vi "sv_Shift and Low Pass Filter (N Ch WDT) with IC.vi"(0 "input signals":waveform(dbl)[](array[waveform]), 1 "reset? (F)":bool, 7 "center":dbl, 9 "decimation factor":i32, 12 "initial conditions":T2 {"filter settings"."filters"."coefficients" format="%.2f"}, 13 "new dt":dbl) -> (4 "enveloped signals":waveform(dbl)[](array[waveform]), 14 "final conditions":T2 {"filter settings"."filters"."coefficients" format="%.2f"})   [LabVIEW 2017, in "SoundVib_FaultAnalysis.lvlib"]
uses:
  <vilib>/addons/Sound and Vibration/Order Analysis/Fault Analysis/SoundVib_FaultAnalysis.lvlib
  <vilib>/addons/_NISVFA/_Shared subVIs/Controls/OAT Decimation Filter.ctl
  <vilib>/addons/Sound and Vibration/Order Analysis/Resample Order Tracking/SubVIs/OAT Frequency Shift (Mixer).vi
  <vilib>/addons/Sound and Vibration/Order Analysis/Resample Order Tracking/SubVIs/oa_Decimation with CIC and Compensation Filter.vi
  <vilib>/addons/Sound and Vibration/Order Analysis/Fault Analysis/SubVIs/oa_Demodulation Initial States (1 Channel).vi
  <vilib>/addons/Sound and Vibration/Order Analysis/Adv Resampling/OAT Single Stage Decimation with IC.vi
  <vilib>/addons/Sound and Vibration/Order Analysis/Resample Order Tracking/SubVIs/OAT CIC Decimation.vi
  <vilib>/addons/Sound and Vibration/Order Analysis/Resample Order Tracking/SubVIs/oa_Interpolate Zeros Between Samples.vi
  <vilib>/addons/Sound and Vibration/Order Analysis/Resample Order Tracking/SubVIs/oa_Calculate Delay of CIC Decimation Interpolation Filter.vi
  <vilib>/addons/Sound and Vibration/Order Analysis/Resample Order Tracking/SubVIs/oa_Create CIC Compensation Filter.vi
  <vilib>/addons/Sound and Vibration/Order Analysis/Resample Order Tracking/SubVIs/oa_Create CIC LP Truncation Filter.vi
  <vilib>/addons/Sound and Vibration/Order Analysis/Resample Order Tracking/SoundVib_Resampling.lvlib
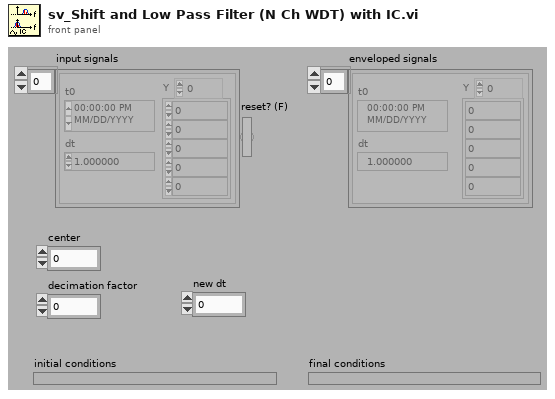
[diagram p1: front panel]
types:
  T1 = typedef "OAT Decimation Filter.ctl" = cluster{"coefficients":dbl[], "factor":i32}
  T2 = cluster{"filter settings":cluster{"CIC Settings":cluster{"Numeric":i32, i32, i32}, "filters":T1[], "delay":i32, "interpolation factor":i32}, "filter states":cluster{"t0":dbl, "phase":dbl, "real filter state":cluster{cluster{dbl[]}, cluster{dbl[]}[]}, "imaginary filter state":cluster{cluster{dbl[]}, cluster{dbl[]}[]}, "delay":i32}[], "reset pending":bool}
  T3 = cluster{"t0":dbl, "phase":dbl, "real filter state":cluster{cluster{dbl[]}, cluster{dbl[]}[]}, "imaginary filter state":cluster{cluster{dbl[]}, cluster{dbl[]}[]}, "delay":i32}[]
  T4 = cluster{"t0":dbl, "phase":dbl, "real filter state":cluster{cluster{dbl[]}, cluster{dbl[]}[]}, "imaginary filter state":cluster{cluster{dbl[]}, cluster{dbl[]}[]}, "delay":i32}
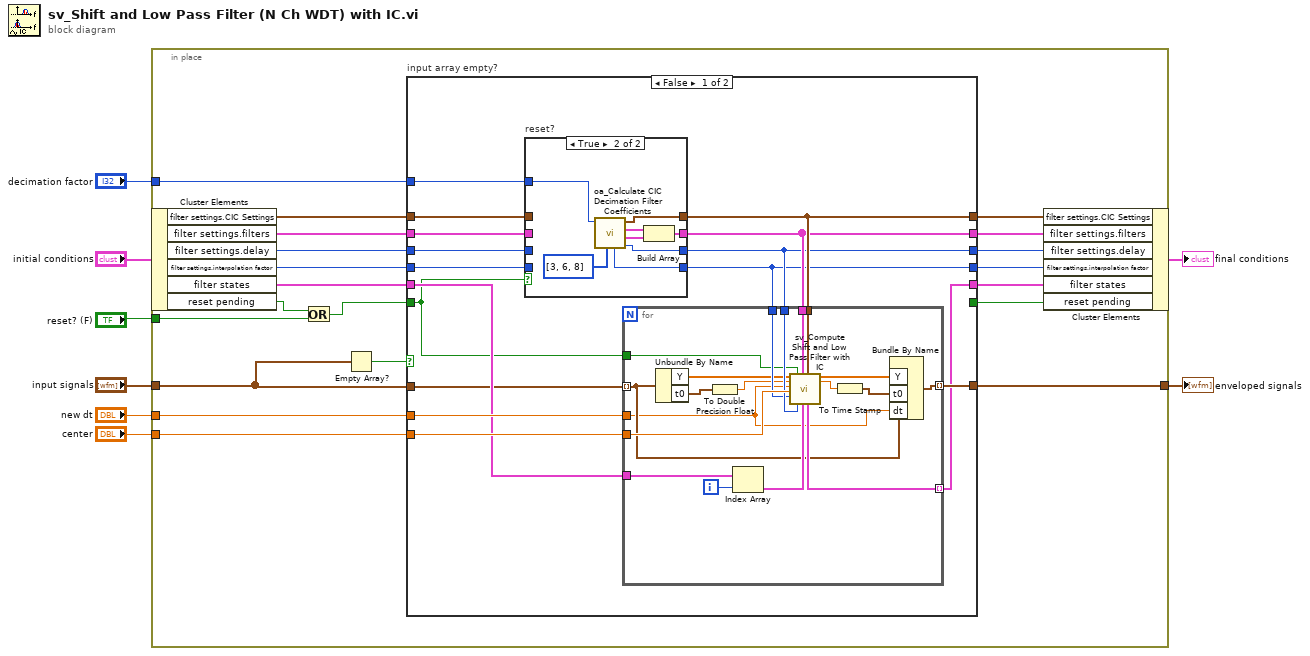
[diagram p0: block diagram]
diagram:
  n1 = in-place {
    in-place-border: "input signals" -> [w9]
    in-place-border: "decimation factor" -> [w28]
    in-place-border: "center" -> [w27]
    in-place-border: "new dt" -> [w26]
    in-place-border: "reset? (F)" -> [w13]
    in-place-border: [w25] -> w1
    n2 = in-place-cluster #1("initial conditions") -> ("filter settings.CIC Settings"=w22:cluster{"Numeric":i32, i32, i32}, "filter settings.filters"=w21:T1[], "filter settings.delay"=w20:i32, "filter settings.interpolation factor"=w19:i32, "filter states"=w24:T3, "reset pending"=w14:bool)
    n3 = Or(x=w14, y=w13) -> (x .or. y?=w12:bool)
    n4 = Empty Array?(array=w9) -> (empty?=w11:bool)
    n5 = case "input array empty?" shown="False" w11 {
      tunnel: w28 -> [w44 _]
      tunnel: w27 -> [w43 _]
      tunnel: w26 -> [w42 _]
      tunnel: [w41 w76] -> w25
      tunnel: w24 -> [w40 w77]
      tunnel: [w39 w77] -> w23
      tunnel: w22 -> [w38 w81]
      tunnel: w21 -> [w37 w80]
      tunnel: w20 -> [w36 w79]
      tunnel: w19 -> [w35 w78]
      tunnel: [w34 w81] -> w18
      tunnel: [w33 w80] -> w17
      tunnel: [w32 w79] -> w16
      tunnel: [w31 w78] -> w15
      tunnel: w12 -> [w30 w82]
      tunnel: [_ w82] -> w10
      tunnel: w9 -> [w29 w76]
      frame False {
        n6 = case "reset?" shown="True" w30 {
          tunnel: [w67 w75] -> w34
          tunnel: [w66 w72] -> w33
          tunnel: [w64 w71] -> w31
          tunnel: [w65 w70] -> w32
          tunnel: w44 -> [_ w69]
          tunnel: w38 -> [w67 _]
          tunnel: w37 -> [w66 _]
          tunnel: w36 -> [w65 _]
          tunnel: w35 -> [w64 _]
          frame False {
          }
          frame True {
            n7 = call <vilib>:"oa_Calculate CIC Decimation Filter Coefficients.vi"("CIC stages"=i32[] [3, 6, 8], "decimation/interpolation factor"=w69) -> ("delay"=w70:i32, "lp filter settings"=w73:T1, "compensation filter settings"=w74:T1, "CIC Settings"=w75:cluster{"Numeric":i32, i32, i32}, "interpolation factor"=w71:i32)  [unwired: 5 in]
            n8 = Build Array(w74, w73) -> (w72:T1[])
          }
        }
        n9 = for {
          tunnel: w43 -> [w63]
          tunnel: w42 -> [w50]
          tunnel: [w47] -> w41 mode=indexing
          tunnel: w40 -> [w58]
          tunnel: [w62] -> w39 mode=indexing
          tunnel: w34 -> [w45]
          tunnel: w33 -> [w46]
          tunnel: w32 -> [w61]
          tunnel: w31 -> [w60]
          tunnel: w30 -> [w59]
          tunnel: w29 -> [w54] mode=indexing
          i -> [w57]
          n10 = Unbundle By Name(w54) -> ("Y"=w55:dbl[], "t0"=w52:timestamp)
          n11 = To Double Precision Float(number=w52) -> (double precision float=w51:dbl)
          n12 = Index Array(array=w58, index=w57) -> (element=w56:T4)
          n13 = call <vilib>:"sv_Compute Shift and Low Pass Filter with IC.vi"("input signal"=w55, "t0"=w51, "new dt"=w50, "center"=w63, "interpolation factor"=w60, "reset? (F)"=w59, "delay"=w61, "filters"=w46, "initial conditions"=w56, "CIC settings"=w45) -> ("final conditions"=w62:T4, "enveloped signal"=w53:dbl[], "t0 out"=w49:dbl)  [unwired: 6 in, 1 out]
          n14 = To Time Stamp(1:w49) -> (0:w48:timestamp)
          n15 = Bundle By Name(cluster=w54, "Y"=w53, "t0"=w48, "dt"=w50) -> (w47:waveform(dbl))
        }
      }
      frame True {
      }
    }
    n16 = in-place-cluster #1("filter settings.CIC Settings"=w18, "filter settings.filters"=w17, "filter settings.delay"=w16, "filter settings.interpolation factor"=w15, "filter states"=w23, "reset pending"=w10) -> (→"final conditions":T2)
  }
  "enveloped signals" <- w1
